vi "GVEncoder.vi"() -> ()   [LabVIEW 2016]
panel:
  in  "CounterReset 7":fxp<+/-,32,32>
  in  "EncdTicks/Cnt 7":fxp<+,32,32>
  in  "EncdPos 7":fxp<+/-,32,32>
  in  "EncdDir 7":fxp<+/-,2,2>
  in  "EncdCnt 7":fxp<+/-,32,32>
  in  "CounterReset 6":fxp<+/-,32,32>
  in  "EncdTicks/Cnt 6":fxp<+,32,32>
  in  "EncdPos 6":fxp<+/-,32,32>
  in  "EncdDir 6":fxp<+/-,2,2>
  in  "EncdCnt 6":fxp<+/-,32,32>
  in  "CounterReset 5":fxp<+/-,32,32>
  in  "EncdTicks/Cnt 5":fxp<+,32,32>
  in  "EncdPos 5":fxp<+/-,32,32>
  in  "EncdDir 5":fxp<+/-,2,2>
  in  "EncdCnt 5":fxp<+/-,32,32>
  in  "CounterReset 4":fxp<+/-,32,32>
  in  "EncdTicks/Cnt 4":fxp<+,32,32>
  in  "EncdPos 4":fxp<+/-,32,32>
  in  "EncdDir 4":fxp<+/-,2,2>
  in  "EncdCnt 4":fxp<+/-,32,32>
  in  "CounterReset 3":fxp<+/-,32,32>
  in  "CounterReset 2":fxp<+/-,32,32>
  in  "CounterReset 1":fxp<+/-,32,32>
  in  "EncdTicks/Cnt 3":fxp<+,32,32>
  in  "EncdPos 3":fxp<+/-,32,32>
  in  "EncdDir 3":fxp<+/-,2,2>
  in  "EncdCnt 3":fxp<+/-,32,32>
  in  "EncdTicks/Cnt 2":fxp<+,32,32>
  in  "EncdPos 2":fxp<+/-,32,32>
  in  "EncdDir 2":fxp<+/-,2,2>
  in  "EncdCnt 2":fxp<+/-,32,32>
  in  "EncdTicks/Cnt 1":fxp<+,32,32>
  in  "EncdPos 1":fxp<+/-,32,32>
  in  "EncdDir 1":fxp<+/-,2,2>
  in  "EncdCnt 1":fxp<+/-,32,32>
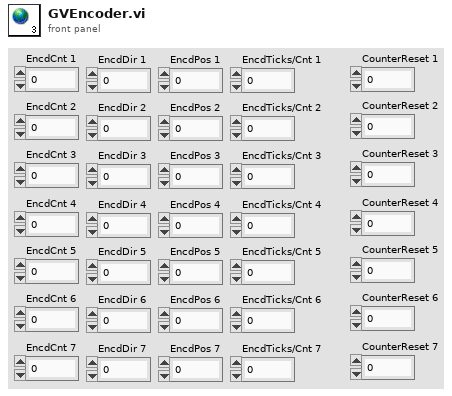
[diagram p1: front panel]
diagram:
